vi "Player Info.vi"(8 "Victory Speech":string="All your base are belong to us!!", 9 "Name":string, 11 "Scout in":refnum<class "Scout.lvclass">) -> (3 "Scout out":refnum<class "Scout.lvclass">)   [LabVIEW 2015, in "Scout.lvclass"]
uses:
  Scout.lvclass
  Formics/Formics.lvclass
panel:
  # "Set default values for these two string controls"
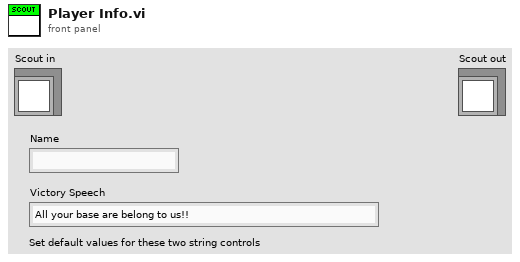
[diagram p1: front panel]
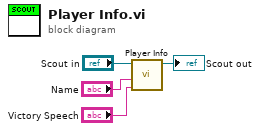
[diagram p0: block diagram]
diagram:
  n1 = call-parent "Player Info.vi"("Victory Speech"="Victory Speech", "Name"="Name", "Formics in"="Scout in") -> ("Formics out"=→"Scout out":refnum<class "Scout.lvclass">)  [unwired: 8 in]
